vi "ExtractControlRefsFromVi.vi"(7 "Indicators":bool, 8 "error in (no error)":errorcluster, 10 "ShowAllControls?":bool, 11 "VI in":refnum<vi>) -> (0 "error out":errorcluster, 3 "Controls":T1[](array[typedef]))   [LabVIEW 2020, in "ContextHelpEditor.lvlib"]
uses:
  ContextHelpEditor.lvlib
  ControlRef--cluster.ctl
  <vilib>/picture/picture.llb/imagedata.ctl
  <vilib>/Utility/traverseref.llb/VI Scripting - Traverse.lvlib
  <vilib>/Utility/traverseref.llb/TRef TravTarget.ctl
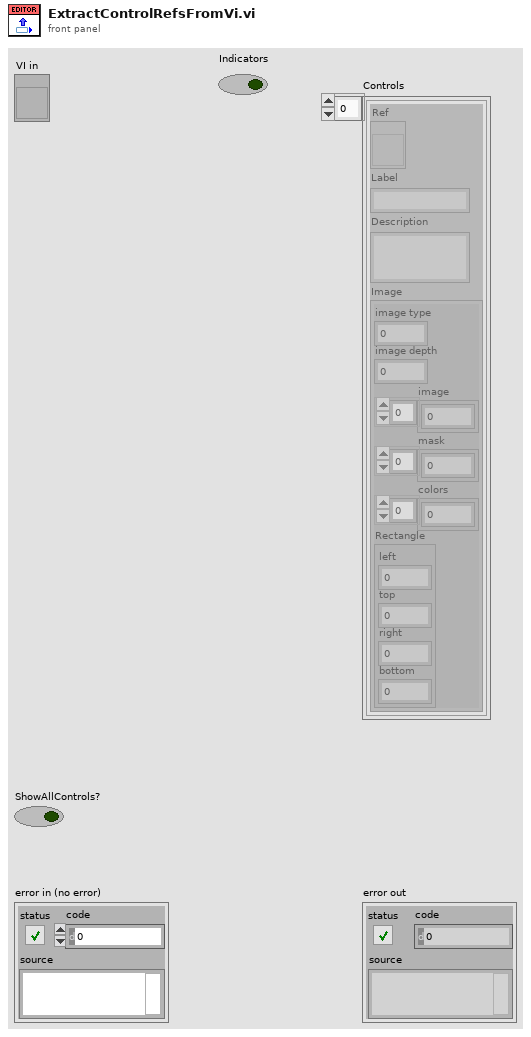
[diagram p1: front panel]
types:
  T1 = typedef "ContextHelpEditor.lvlib/ControlRef--cluster.ctl" = cluster{"Ref":refnum<vi>, "Label":string, "Description":string, "Image":T2}
  T2 = typedef "imagedata.ctl" = cluster{"image type":i32, "image depth":i32, "image":u8[], "mask":u8[], "colors":u32[], "Rectangle":cluster{"left":i16, "top":i16, "right":i16, "bottom":i16}}
  T3 = typedef "TRef TravTarget.ctl" = enum16{"FP", "BD", "Other"}
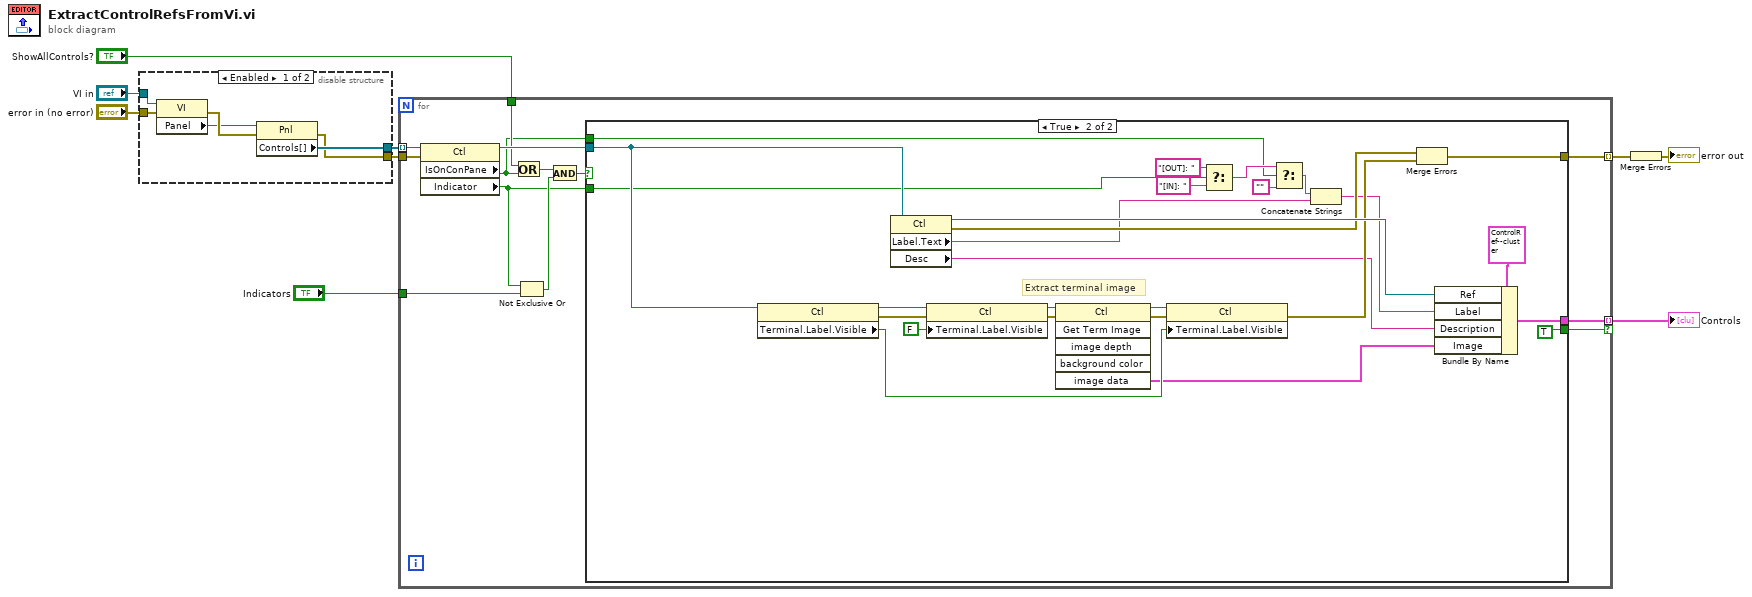
[diagram p0: block diagram]
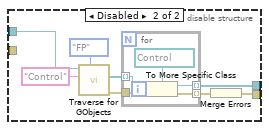
[diagram p2: hidden frame]
diagram:
  n1 = disable-structure shown="Enabled" {
    disable-tunnel: [w15 w19] -> w9
    disable-tunnel: "VI in" -> [w14 w22]
    disable-tunnel: "error in (no error)" -> [w13 _]
    disable-tunnel: [w11 w16] -> w6
    frame Enabled {
      n2 = property class="VI"(reference=w14, error in=w13) -> (error out=w12:errorcluster, "Panel"=w10:refnum<vi>)  [unwired: 1 out]
      n3 = property class="Pnl"(reference=w10, error in=w12) -> (error out=w11:errorcluster, "Controls[]"=w15:refnum<vi>[])  [unwired: 1 out]
    }
    frame Disabled {
      n4 = call <vilib>:"Traverse for GObjects.vi"("Traverse Target"=TRef_TravTarget."FP", "Class Name"="Control", "VI Refnum"=w22) -> ("error out"=w18:errorcluster, "References"=w20:refnum<vi>[])  [unwired: 5 in, 2 out]
      n5 = for {
        tunnel: w20 -> [w28] mode=indexing
        tunnel: [w27] -> w19 mode=indexing
        tunnel: w18 -> [w25]
        tunnel: [w24] -> w17 mode=indexing
        n6 = To More Specific Class(target class=refnum<vi> refnum, reference=w28, error in=w25) -> (specific class reference=w27:refnum<vi>, error out=w24:errorcluster)
      }
      n7 = Merge Errors(w17) -> (w16:errorcluster)
    }
  }
  n8 = for {
    tunnel: w9 -> [w41] mode=indexing
    tunnel: [w38] -> w5 mode=indexing if=w33
    tunnel: "Indicators" -> [w35]
    tunnel: "ShowAllControls?" -> [w31]
    tunnel: w6 -> [w39]
    tunnel: [w37] -> w4 mode=indexing
    n9 = property class="Ctl"(reference=w41, error in=w39) -> (reference out=w40:refnum<vi>, "IsOnConPane"=w29:bool, "Indicator"=w30:bool)  [unwired: 1 out]
    n10 = Or(x=w31, y=w29) -> (x .or. y?=w32:bool)
    n11 = Not Exclusive Or(1:w35, 2:w30) -> (0:w34:bool)
    n12 = And(x=w32, y=w34) -> (x .and. y?=w36:bool)
    n13 = case shown="True" w36 {
      tunnel: w40 -> [_ w54]
      tunnel: [_ w66] -> w38
      tunnel: [_ w63] -> w37
      tunnel: [_ TRUE] -> w33
      tunnel: w30 -> [_ w43]
      tunnel: w29 -> [_ w42]
      frame False {
      }
      frame True {
        # "Extract terminal image"
        n14 = property class="Ctl"(reference=w54) -> (reference out=w55:refnum<vi>, error out=w56:errorcluster, "Terminal.Label.Visible"=w53:bool)  [unwired: 1 in]
        n15 = property class="Ctl"(reference=w54) -> (reference out=w67:refnum<vi>, error out=w64:errorcluster, "Label.Text"=w52:string, "Desc"=w45:string)  [unwired: 1 in]
        n16 = property class="Ctl"(reference=w55, error in=w56, "Terminal.Label.Visible"=FALSE) -> (reference out=w60:refnum<vi>, error out=w61:errorcluster)
        n17 = invoke class="Ctl" method="Get Term Image"(reference=w60, error in=w61) -> (reference out=w57:refnum<vi>, error out=w65:errorcluster, "image data"=w44:T2)  [unwired: 4 in, 3 out]
        n18 = property class="Ctl"(reference=w57, error in=w65, "Terminal.Label.Visible"=w53) -> (error out=w58:errorcluster)  [unwired: 1 out]
        n19 = Select(t="[OUT]: ", s=w43, f="[IN]: ") -> (s? t:f=w48:string)
        n20 = Select(t=w48, s=w42, f="") -> (s? t:f=w47:string)
        n21 = Concatenate Strings(w47, w52) -> (w51:string)
        n22 = Merge Errors(w64, w58) -> (w63:errorcluster)
        n23 = Bundle By Name(cluster=T1 {"Ref"=refnum, "Label"="", "Description"="", "Image"={"image type"=0, "image depth"=0, "image"=[], "mask"=[], "colors"=[], "Rectangle"={"left"=0, "top"=0, "right"=0, "bottom"=0}}} ("ControlRef"), "Ref"=w67, "Label"=w51, "Description"=w45, "Image"=w44) -> (w66:T1)
      }
    }
  }
  "Controls" <- w5
  n24 = Merge Errors(w4) -> (→"error out":errorcluster)
